vi "CreateHTML.vi"(0 "reference in":refnum<class "WebFrontPanel.lvclass">, 5 "error in (no error)":errorcluster, 7 "Refresh rate (250ms)":i32=250) -> (12 "Name":string, 14 "reference out":refnum<class "WebFrontPanel.lvclass">, 15 "HTML":string, 16 "js":string, 19 "error out":errorcluster)   [LabVIEW 2014, in "WebFrontPanel.lvclass"]
uses:
  WebFrontPanel.lvclass
  Controls/HTMLTemplateFill.ctl
  Controls/JSTemplateFill.ctl
  <userlib>/_OpenG.lib/array/array.llb/Remove Duplicates from 1D Array (String)__ogtk.vi
  Object_class/Object.lvclass
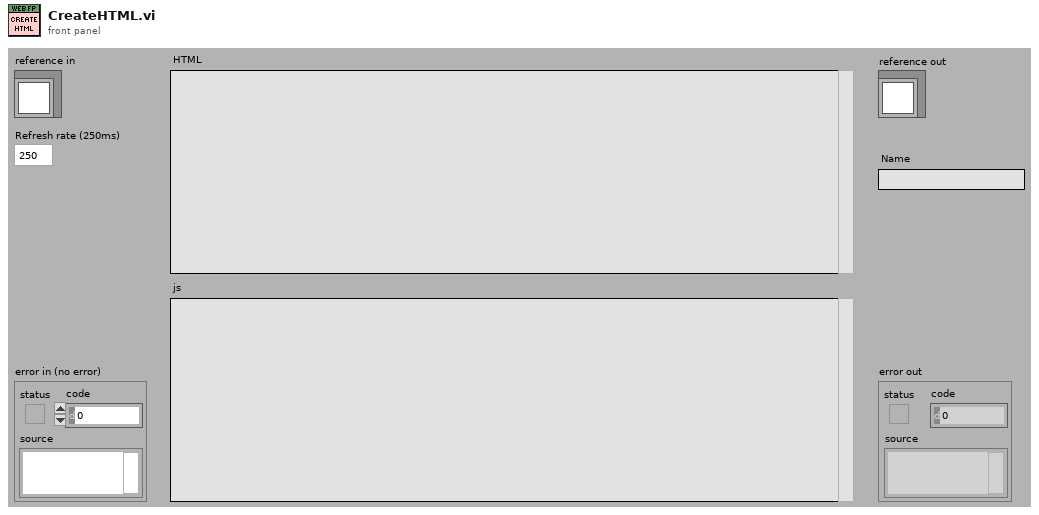
[diagram p1: front panel]
types:
  T1 = typedef "WebFrontPanel.lvclass/JSTemplateFill.ctl" = cluster{"Page Name":string, "js varibles":string, "Code for controls":string, "Code for indicators":string, "Refresh rate (ms)":i32}
  T2 = typedef "WebFrontPanel.lvclass/HTMLTemplateFill.ctl" = cluster{"Page Name":string, "Script dependencies":string, "Body width (px)":i32, "Body height (px)":i32, "Background Colour":u32, "HTML elements":string}
  T3 = typedef "WebFrontPanel.lvclass/ObjectAttributes.ctl" = cluster{"VI Name":string, "VI Reference":refnum<vi>, "Controls":refnum<class "Object.lvclass">[], "Indicators":refnum<class "Object.lvclass">[], "Decorations":refnum<class "Object.lvclass">[]}
  T4 = typedef "LVRectTypeDef.ctl" = cluster{"Left":i16, "Top":i16, "Right":i16, "Bottom":i16}
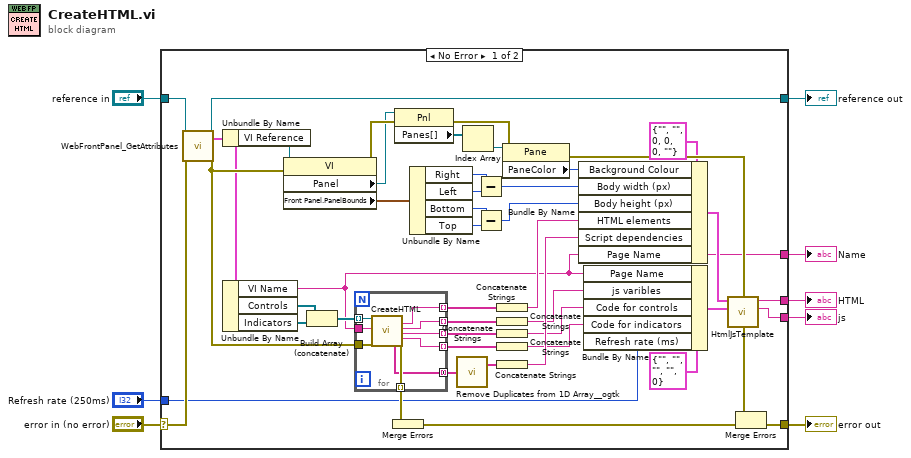
[diagram p0: block diagram]
diagram:
  n1 = case shown="No Error" "error in (no error)" {
    selector: "error in (no error)" -> [w53 w64]
    tunnel: [w48 w64] -> w7
    tunnel: [w45 w63] -> w5
    tunnel: "reference in" -> [w46 w63]
    tunnel: [w26 _] -> w3
    tunnel: "Refresh rate (250ms)" -> [w9 _]
    tunnel: [w10 _] -> w2
    tunnel: [w12 _] -> w1
    frame No Error {
      n2 = call "WebFrontPanel_GetAttributes.vi"("reference in"=w46, "error in (no error)"=w53) -> ("reference out"=w45:refnum<class "WebFrontPanel.lvclass">, "Data"=w30:T3, "error out"=w51:errorcluster)  [unwired: 14 in, 1 out]
      n3 = Unbundle By Name(w30) -> ("VI Reference"=w34:refnum<vi>)
      n4 = Unbundle By Name(w30) -> ("VI Name"=w12:string, "Controls"=w29:refnum<class "Object.lvclass">[], "Indicators"=w28:refnum<class "Object.lvclass">[])
      n5 = property class="VI"(reference=w34, error in=w51) -> (error out=w50:errorcluster, "Panel"=w19:refnum<vi>, "Front Panel.PanelBounds"=w39:T4)  [unwired: 1 out]
      n6 = Build Array (concatenate)(w29, w28) -> (w31:refnum<class "Object.lvclass">[])
      n7 = for {
        tunnel: w31 -> [w60] mode=indexing
        tunnel: [w59] -> w44 mode=indexing
        tunnel: [w58] -> w43 mode=indexing
        tunnel: [w57] -> w42 mode=indexing
        tunnel: [w56] -> w41 mode=concatenating
        tunnel: w51 -> [w62]
        tunnel: [w61] -> w33 mode=indexing
        tunnel: [w55] -> w32 mode=indexing
        tunnel: w12 -> [w54]
        n8 = call-dynamic "CreateHTML.vi"("reference in"=w60, "VI Name"=w54, "error in (no error)"=w62) -> ("script dependencies"=w56:string[], "HTML"=w59:string, "js variables"=w58:string, "js code for controls"=w57:string, "js code for indicators"=w55:string, "error out"=w61:errorcluster)  [unwired: 10 in, 1 out]
      }
      n9 = Merge Errors(w33) -> (w52:errorcluster)
      n10 = property class="Pnl"(reference=w19, error in=w50) -> (error out=w49:errorcluster, "Panes[]"=w21:refnum<vi>[])  [unwired: 1 out]
      n11 = Unbundle By Name(w39) -> ("Right"=w38:i16, "Left"=w37:i16, "Bottom"=w36:i16, "Top"=w35:i16)
      n12 = call-poly <userlib>:"Remove Duplicates from 1D Array__ogtk.vi"("Input Array"=w41) -> ("Output Array"=w40:string[])  [unwired: 1 out]
      n13 = Index Array(array=w21) -> (element=w20:refnum<vi>)  [unwired: 1 in]
      n14 = Subtract(x=w38, y=w37) -> (x-y=w25:i16)
      n15 = Subtract(x=w36, y=w35) -> (x-y=w24:i16)
      n16 = Concatenate Strings(w44) -> (w23:string)
      n17 = Concatenate Strings(w43) -> (w15:string)
      n18 = Concatenate Strings(w42) -> (w14:string)
      n19 = Concatenate Strings(w32) -> (w13:string)
      n20 = Concatenate Strings(w40) -> (w22:string)
      n21 = property class="Pane"(reference=w20, error in=w49) -> (error out=w47:errorcluster, "PaneColor"=w18:u32)  [unwired: 1 out]
      n22 = Bundle By Name(cluster=T2 {"Page Name"="", "Script dependencies"="", "Body width (px)"=0, "Body height (px)"=0, "Background Colour"=0, "HTML elements"=""} ("HTML"), "Background Colour"=w18, "Body width (px)"=w25, "Body height (px)"=w24, "HTML elements"=w23, "Script dependencies"=w22, "Page Name"=w12) -> (w17:T2)
      n23 = Bundle By Name(cluster=T1 {"Page Name"="", "js varibles"="", "Code for controls"="", "Code for indicators"="", "Refresh rate (ms)"=0} ("js"), "Page Name"=w12, "js varibles"=w15, "Code for controls"=w14, "Code for indicators"=w13, "Refresh rate (ms)"=w9) -> (w11:T1)
      n24 = call "HtmlJsTemplate.vi"("js"=w11, "HTML"=w17) -> ("js out"=w10:string, "HTML out"=w26:string)  [unwired: 8 in]
      n25 = Merge Errors(w47, w52) -> (w48:errorcluster)
    }
    frame Error {
    }
  }
  "error out" <- w7
  "reference out" <- w5
  "HTML" <- w3
  "js" <- w2
  "Name" <- w1
